vi "Step Responsevi.vi"(8 "Number":dbl=50.0 format="%#_13g", 9 "dt, msec":u32=1000, 10 "PV":dbl, 11 "Data In":dbl[][](array[numeric])) -> (2 "Complete Data Acquisition":bool, 3 "Data Out":dbl[][](array[numeric]))   [LabVIEW 2014]
panel:
  out "How many values   were counted":i32
  out "Volume":dbl
  out "Condition on \nSKO\nin progress \n100 times":bool
  out "SKO(i)-SKO(i-1) <= 0,05*SKO(i)?":bool
  out "Mean square deviation":dbl
  out "Среднее значение":dbl
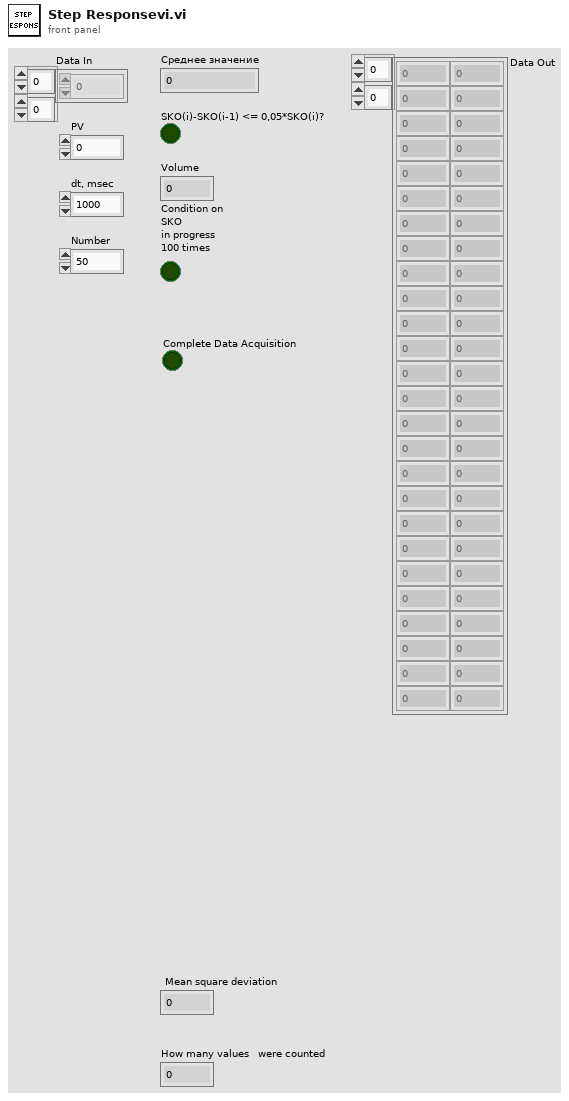
[diagram p1: front panel]
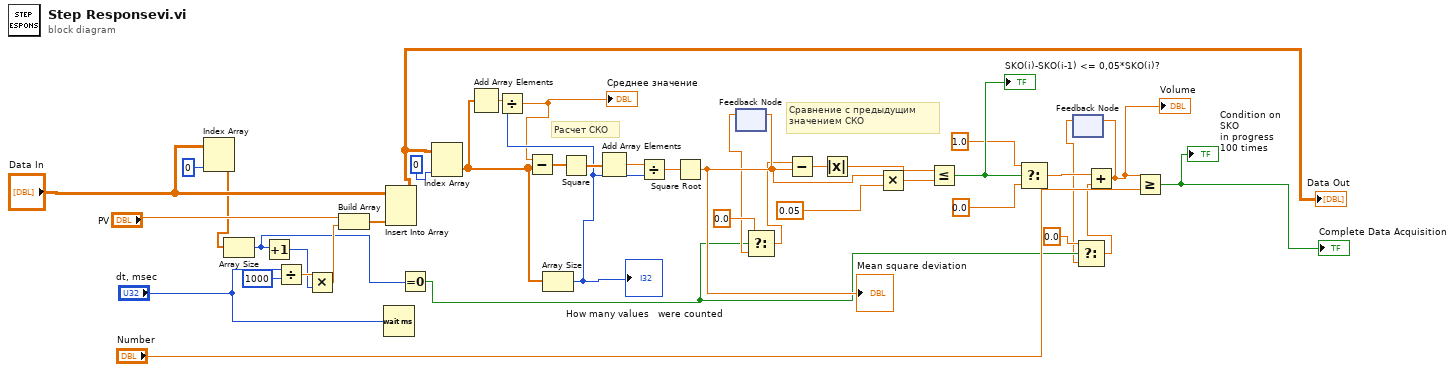
[diagram p0: block diagram]
diagram:
  # "Сравнение с предыдущим \nзначением СКО"
  # "Расчет СКО"
  n1 = Index Array(array="Data In", index (col)=0 ("disabled index (col)")) -> (element=w11:dbl[])  [unwired: 1 in]
  n2 = Array Size(array=w11) -> (size(s)=w9:i32)
  n3 = Increment(x=w9) -> (x+1=w13:i32)
  n4 = Divide(x="dt, msec", y=u32 1000) -> (x/y=w39:dbl)
  n5 = Multiply(x=w39, y=w13) -> (x*y=w38:dbl)
  n6 = Build Array("PV", w38) -> (w36:dbl[])
  n7 = Wait (ms)(milliseconds to wait="dt, msec") -> ()  [unwired: 1 out]
  n8 = Insert Into Array(array="Data In", new element=w36) -> (w40:dbl[][])  [unwired: 2 in]
  "Data Out" <- w40
  n9 = Equal To 0?(x=w9) -> (x = 0?=w5:bool)
  n10 = Index Array(array=w40, index (col)=0 ("index (row)")) -> (element=w17:dbl[])  [unwired: 1 in]
  n11 = Add Array Elements(numeric array=w17) -> (sum=w23:dbl)
  n12 = Array Size(array=w17) -> (size(s)=w22:i32)
  "How many values   were counted" <- w22
  n13 = Divide(x=w23, y=w22) -> (x/y=w21:dbl)
  "Среднее значение" <- w21
  n14 = Subtract(x=w21, y=w17) -> (x-y=w25:dbl[])
  n15 = Square(x=w25) -> (x^2=w24:dbl[])
  n16 = Add Array Elements(numeric array=w24) -> (sum=w35:dbl)
  n17 = Divide(x=w35, y=w22) -> (x/y=w34:dbl)
  n18 = Square Root(x=w34) -> (sqrt(x)=w20:dbl)
  "Mean square deviation" <- w20
  n19 = feedback #1() -> (w7:dbl)  [unwired: 1 in]
  n20 = feedback-in #1(w20) -> ()
  n21 = Select(t=0.0, s=w5, f=w7) -> (s? t:f=w6:dbl)
  n22 = Subtract(x=w6, y=w20) -> (x-y=w33:dbl)
  n23 = Absolute Value(x=w33) -> (abs(x)=w30:dbl)
  n24 = Multiply(x=w20, y=0.05) -> (x*y=w31:dbl)
  n25 = Less Or Equal?(x=w30, y=w31) -> (x <= y?=w28:bool)
  "SKO(i)-SKO(i-1) <= 0,05*SKO(i)?" <- w28
  n26 = Select(t=1.0, s=w28, f=0.0) -> (s? t:f=w19:dbl)
  n27 = feedback #2() -> (w3:dbl)  [unwired: 1 in]
  n28 = Select(t=0.0, s=w5, f=w3) -> (s? t:f=w2:dbl)
  n29 = Add(x=w19, y=w2) -> (x+y=w16:dbl)
  "Volume" <- w16
  n30 = feedback-in #2(w16) -> ()
  n31 = Greater Or Equal?(x=w16, y="Number") -> (x >= y?=→"Condition on \nSKO\nin progress \n100 times" →"Complete Data Acquisition":bool)
